vi "h.DETECTION.GetDetectionSetting.vi"(8 "error in":errorcluster, 10 "Detection Setting Index":u8, 11 "Connection ID":refnum<k5>) -> (0 "error out":errorcluster, 2 "Detection Setting":T1, 3 "Connection ID out":refnum<k5>)   [LabVIEW 2016, in "h.Library.lvlib"]
uses:
  h.Library.lvlib
  h.DETECTION.PeakDetectionPreset.ctl
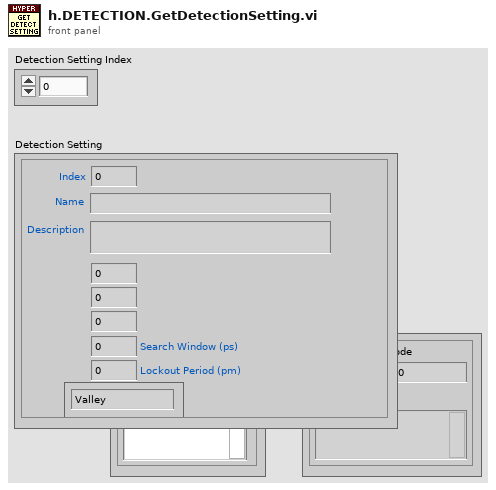
[diagram p1: front panel]
types:
  T1 = typedef "h.Library.lvlib/h.DETECTION.PeakDetectionPreset.ctl" = cluster{"Index":u8, "Name":string, "Description":string, "Detection Mode":enum32{"Valley", "Peak"}, "Averaging Window (pm)":i32, "Peak Width (pm)":i32, "Lockout Period (pm)":i32, "Search Window (ps)":i32, "Threshold Level":i32}
  T2 = enum16{"big-endian, network order", "native, host order", "little-endian"}
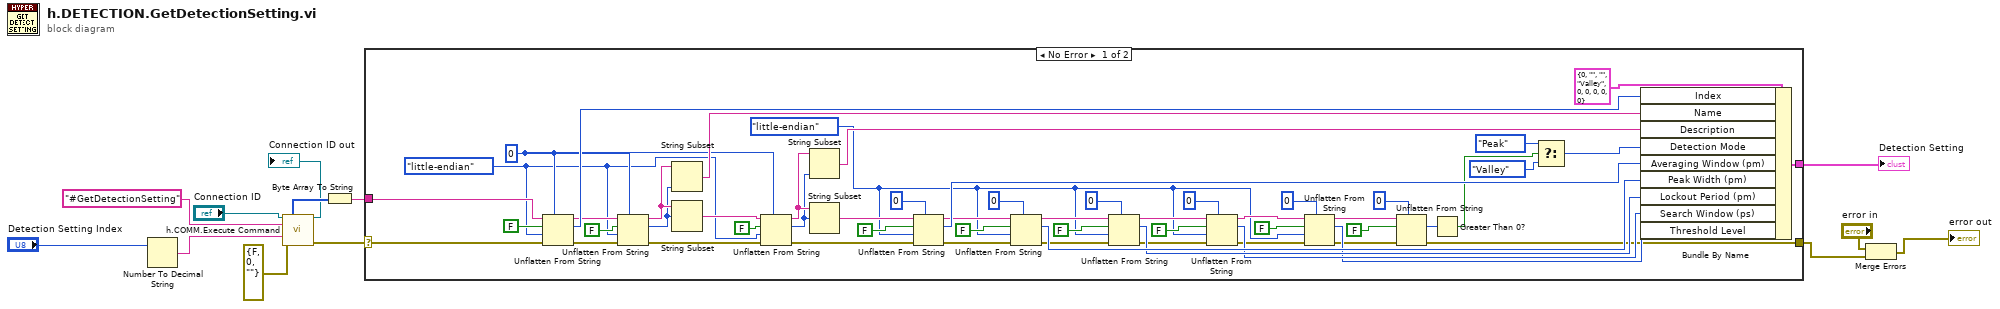
[diagram p0: block diagram]
diagram:
  n1 = Number To Decimal String(number="Detection Setting Index") -> (decimal integer string=w6:string)  [unwired: 1 in]
  n2 = call "h.COMM.Execute Command.vi"("Connection ID"="Connection ID", "Command"="#GetDetectionSetting", "Argument"=w6, "error in"=errorcluster {"status"=FALSE, "code"=0, "source"=""}) -> ("Content"=w11:u8[], "Connection ID out"=→"Connection ID out":refnum<k5>, "error out"=w8:errorcluster)  [unwired: 4 in, 5 out]
  n3 = Byte Array To String(unsigned byte array=w11) -> (string=w10:string)
  n4 = case shown="No Error" w8 {
    selector: w8 -> [w14 w70]
    tunnel: w10 -> [w69 _]
    tunnel: [w26 _] -> w5
    tunnel: [w21 w70] -> w3
    frame No Error {
      w15 = T2."little-endian" ("byte order (0:big-endian, network order)")
      w57 = u8 0
      w55 = T2."little-endian" ("byte order (0:big-endian, network order)")
      n5 = Unflatten From String(type=w57, binary string=w69, data includes array or string size? (T)=FALSE, byte order (0:big-endian, network order)=w55, error in (no error)=w14) -> (rest of the binary string=w64:string, value=w66:u8, error out=w63:errorcluster)
      n6 = Unflatten From String(type=w57, binary string=w64, data includes array or string size? (T)=FALSE, byte order (0:big-endian, network order)=w55, error in (no error)=w63) -> (rest of the binary string=w61:string, value=w60:u8, error out=w58:errorcluster)
      n7 = String Subset(string=w61, length (rest)=w60) -> (substring=w62:string)  [unwired: 1 in]
      n8 = String Subset(string=w61, offset (0)=w60) -> (substring=w56:string)  [unwired: 1 in]
      n9 = Unflatten From String(type=w57, binary string=w56, data includes array or string size? (T)=FALSE, byte order (0:big-endian, network order)=w55, error in (no error)=w58) -> (rest of the binary string=w53:string, value=w52:u8, error out=w49:errorcluster)
      n10 = String Subset(string=w53, length (rest)=w52) -> (substring=w54:string)  [unwired: 1 in]
      n11 = String Subset(string=w53, offset (0)=w52) -> (substring=w50:string)  [unwired: 1 in]
      n12 = Unflatten From String(type=u16 0, binary string=w50, data includes array or string size? (T)=FALSE, byte order (0:big-endian, network order)=w15, error in (no error)=w49) -> (rest of the binary string=w44:string, value=w47:u16, error out=w43:errorcluster)
      n13 = Unflatten From String(type=u16 0, binary string=w44, data includes array or string size? (T)=FALSE, byte order (0:big-endian, network order)=w15, error in (no error)=w43) -> (rest of the binary string=w39:string, value=w42:u16, error out=w38:errorcluster)
      n14 = Unflatten From String(type=u16 0, binary string=w39, data includes array or string size? (T)=FALSE, byte order (0:big-endian, network order)=w15, error in (no error)=w38) -> (rest of the binary string=w33:string, value=w37:u16, error out=w34:errorcluster)
      n15 = Unflatten From String(type=u16 0, binary string=w33, data includes array or string size? (T)=FALSE, byte order (0:big-endian, network order)=w15, error in (no error)=w34) -> (rest of the binary string=w28:string, value=w32:u16, error out=w29:errorcluster)
      n16 = Unflatten From String(type=0, binary string=w28, data includes array or string size? (T)=FALSE, byte order (0:big-endian, network order)=w15, error in (no error)=w29) -> (rest of the binary string=w23:string, value=w27:i32, error out=w22:errorcluster)
      n17 = Unflatten From String(type=u8 0, binary string=w23, data includes array or string size? (T)=FALSE, error in (no error)=w22) -> (value=w19:u8, error out=w21:errorcluster)  [unwired: 1 in, 1 out]
      n18 = Greater Than 0?(x=w19) -> (x > 0?=w20:bool)
      n19 = Select(t=enum32{"Valley", "Peak"}."Peak" ("Detection Mode"), s=w20, f=enum32{"Valley", "Peak"}."Valley" ("Detection Mode")) -> (s? t:f=w16:enum32{"Valley", "Peak"})
      n20 = Bundle By Name(cluster=T1 {"Index"=0, "Name"="", "Description"="", "Detection Mode"=enum."Valley", "Averaging Window (pm)"=0, "Peak Width (pm)"=0, "Lockout Period (pm)"=0, "Search Window (ps)"=0, "Threshold Level"=0} ("Preset"), "Index"=w66, "Name"=w62, "Description"=w54, "Detection Mode"=w16, "Averaging Window (pm)"=w47, "Peak Width (pm)"=w42, "Lockout Period (pm)"=w37, "Search Window (ps)"=w32, "Threshold Level"=w27) -> (w26:T1)
    }
    frame Error {
    }
  }
  "Detection Setting" <- w5
  n21 = Merge Errors("error in", w3) -> (→"error out":errorcluster)
